vi "Clear Faults.vi"(8 "error in (no error)":errorcluster, 10 "CAN Offset":u32=160 format="%x", 11 "interface object in":refnum<k20>) -> (0 "error out":errorcluster, 3 "interface object out":refnum<k20>)   [LabVIEW 2014]
uses:
  <vilib>/RioEmbeddedCAN/RioEmbeddedCAN.llb/CANWrite.vi
  <vilib>/RioEmbeddedCAN/RioEmbeddedCAN.llb/CANWait.vi
  <vilib>/RioEmbeddedCAN/RioEmbeddedCAN.llb/CANWaitTransmitComplete.vi
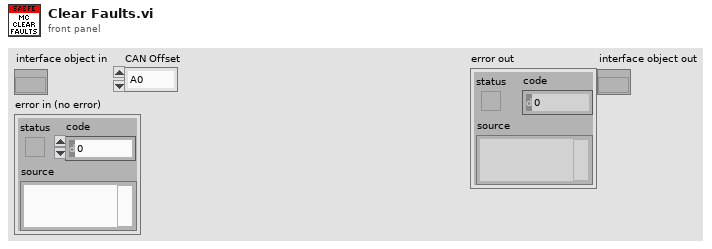
[diagram p1: front panel]
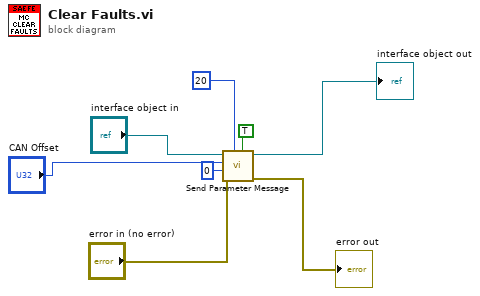
[diagram p0: block diagram]
diagram:
  n1 = call "Send Parameter Message.vi"("Write?"=TRUE, "Param Address"=i16 20, "error in (no error)"="error in (no error)", "Data"=i16 0, "CAN Offset"="CAN Offset", "interface object in"="interface object in") -> ("error out"=→"error out":errorcluster, "interface object out"=→"interface object out":refnum<k20>)  [unwired: 4 in]
